vi "loop.vi"() -> ()   [LabVIEW 2017]
panel:
  out "Iteration":i32
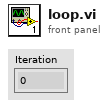
[diagram p1: front panel]
types:
  T1 = cluster{"Boolean array[0]":bool, "Boolean array[1]":bool, "Boolean array[2]":bool, "Boolean array[3]":bool, "Boolean array[4]":bool, "Boolean array[5]":bool}
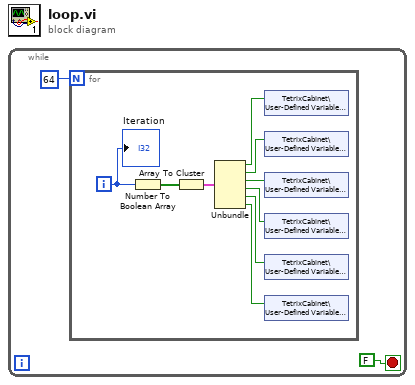
[diagram p0: block diagram]
diagram:
  n1 = while {
    stop <- FALSE stop-if-true
    n2 = for {
      N: 64 -> [_]
      i -> [w9]
      n3 = Number To Boolean Array(number=w9) -> (Boolean array=w11:bool[])
      n4 = Array To Cluster(array=w11) -> (cluster=w10:T1)
      n5 = Unbundle(w10) -> ("Boolean array[0]"=w8:bool, "Boolean array[1]"=w7:bool, "Boolean array[2]"=w6:bool, "Boolean array[3]"=w5:bool, "Boolean array[4]"=w4:bool, "Boolean array[5]"=w3:bool)
      n6 = shared-variable "TetrixCabinet\\User-Defined Variables\\Input_1"(w8) -> ()  [unwired: 1 in, 1 out]
      n7 = shared-variable "TetrixCabinet\\User-Defined Variables\\Input_2"(w7) -> ()  [unwired: 1 in, 1 out]
      n8 = shared-variable "TetrixCabinet\\User-Defined Variables\\Input_3"(w6) -> ()  [unwired: 1 in, 1 out]
      n9 = shared-variable "TetrixCabinet\\User-Defined Variables\\Input_4"(w5) -> ()  [unwired: 1 in, 1 out]
      n10 = shared-variable "TetrixCabinet\\User-Defined Variables\\Input_5"(w4) -> ()  [unwired: 1 in, 1 out]
      n11 = shared-variable "TetrixCabinet\\User-Defined Variables\\Input_6"(w3) -> ()  [unwired: 1 in, 1 out]
      "Iteration" <- w9
    }
  }
